vi "Fade In Core.vi"(6 "Fade Time":u32, 8 "error in (no error)":errorcluster, 9 "End Transparency":u8, 10 "Start Transparency":u8, 11 "VI in":refnum<vi>) -> (0 "error out":errorcluster, 3 "VI out":refnum<vi>)   [LabVIEW 2023, in "Dialog.lvclass"]
doc: "<b> </b> <b> </b>\n©2016 Q Software Innovations, LLC (QSI)\nwritten by Quentin Alldredge\nproduced in LabVIEW 2015\n\nsupport@qsoftwareinnovations.com\nwww.qsoftwareinnovations.com\n\nAll rights reserved.\n\nRedistribution and use in source and binary forms, with or without modification, are permitted provided that the following conditions are met:\n\n * Redistributions of source code must retain the above copyright notice, this list of conditions and the following disclaimer.\n * Redistributions in binary form must reproduce the above copyright notice, this list of conditions and the following disclaimer in the documentation and/or other materials provided with the distribution.\n * Neither the name of Q Software Innovations, LLC. nor the names of its contributors may be used to endorse or promote products derived from this software without specific prior written permission.\n\nTHIS SOFTWARE IS PROVIDED BY THE COPYRIGHT HOLDERS AND CONTRIBUTORS \"AS IS\" AND ANY EXPRESS OR IMPLIED WARRANTIES, INCLUDING, BUT NOT LIMITED TO, THE IMPLIED WARRANTIES OF MERCHANTABILITY AND FITNESS FOR A PARTICULAR PURPOSE ARE DISCLAIMED. IN NO EVENT SHALL THE COPYRIGHT OWNER OR CONTRIBUTORS BE LIABLE FOR ANY DIRECT, INDIRECT, INCIDENTAL, SPECIAL, EXEMPLARY, OR CONSEQUENTIAL DAMAGES (INCLUDING, BUT NOT LIMITED TO, PROCUREMENT OF SUBSTITUTE GOODS OR SERVICES; LOSS OF USE, DATA, OR PROFITS; OR BUSINESS INTERRUPTION) HOWEVER CAUSED AND ON ANY THEORY OF LIABILITY, WHETHER IN CONTRACT, STRICT LIABILITY, OR TORT (INCLUDING NEGLIGENCE OR OTHERWISE) ARISING IN ANY WAY OUT OF THE USE OF THIS SOFTWARE, EVEN IF ADVISED OF THE POSSIBILITY OF SUCH DAMAGE."
uses:
  Dialog.lvclass
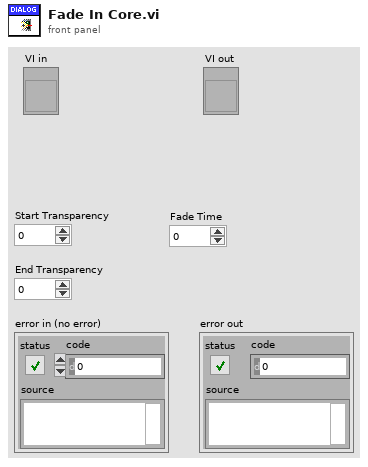
[diagram p1: front panel]
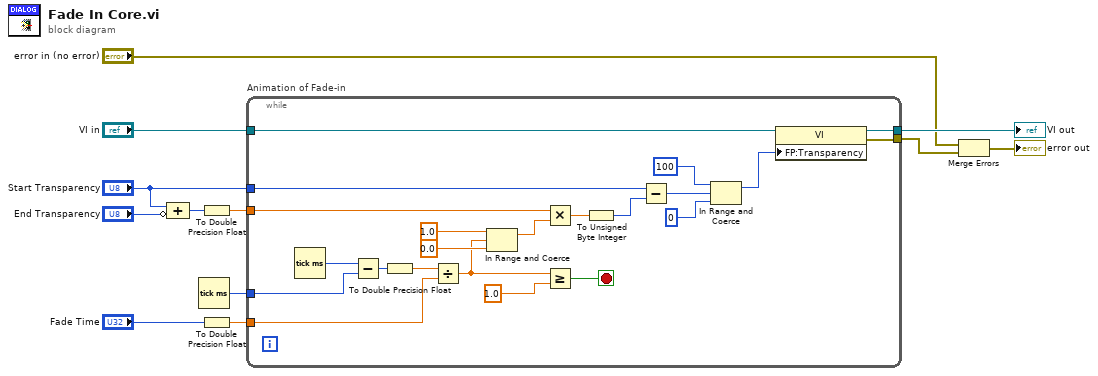
[diagram p0: block diagram]
diagram:
  n1 = Compound Arithmetic op=ADD("Start Transparency", invert "End Transparency") -> (w4:u8)
  n2 = Tick Count (ms)() -> (millisecond timer value=w9:u32)
  n3 = To Double Precision Float(number=w4) -> (double precision float=w11:dbl)
  n4 = To Double Precision Float(number="Fade Time") -> (double precision float=w12:dbl)
  n5 = while "Animation of Fade-in" {
    tunnel: "VI in" -> [w34]
    tunnel: w11 -> [w26]
    tunnel: "Start Transparency" -> [w33]
    tunnel: w9 -> [w30]
    tunnel: [w18] -> w7
    tunnel: [w17] -> w6
    tunnel: w12 -> [w16]
    stop <- w27 stop-if-true
    n6 = Tick Count (ms)() -> (millisecond timer value=w31:u32)
    n7 = Subtract(x=w31, y=w30) -> (x-y=w29:u32)
    n8 = To Double Precision Float(number=w29) -> (double precision float=w21:dbl)
    n9 = Divide(x=w21, y=w16) -> (x/y=w20:dbl)
    n10 = In Range and Coerce(upper limit=1.0, x=w20, lower limit=0.0) -> (coerced(x)=w24:dbl)  [unwired: 1 out]
    n11 = Multiply(x=w26, y=w24) -> (x*y=w25:dbl)
    n12 = Greater Or Equal?(x=w20, y=1.0) -> (x >= y?=w27:bool)
    n13 = To Unsigned Byte Integer(number=w25) -> (unsigned 8bit integer=w19:u8)
    n14 = Subtract(x=w33, y=w19) -> (x-y=w32:u8)
    n15 = In Range and Coerce(upper limit=u8 100, x=w32, lower limit=u8 0) -> (coerced(x)=w15:u8)  [unwired: 1 out]
    n16 = property on="Property Node" class="VI"(reference=w34, "FP:Transparency"=w15) -> (reference out=w18:refnum<vi>, error out=w17:errorcluster)  [unwired: 1 in]
  }
  "VI out" <- w7
  n17 = Merge Errors("error in (no error)", w6) -> (→"error out":errorcluster)
